vi "Drive Train Global.vi"() -> ()   [LabVIEW 2018]
panel:
  in  "Robot Slow Threshold":dbl=25.0
  in  "Robot Slow?":bool=TRUE
  in  "Robot Stopped?":bool=TRUE
  in  "Reset Field Position":bool
  in  "Wheel Angle Offsets Practice Bot":T1={"FrontLeft"=-114.2, "FrontRight"=-153.9, "BackLeft"=-23.0, "BackRight"=-19.1}
  in  "Angle Locking to":dbl=540.0
  in  "Angle to Lock To":dbl=180.0
  out "Lock to Angle":bool
  out "Robot Centric":bool
  in  "Don't Turn While Translate PID Gains":T2 {"derivative time (Td, min)" format="%.3f"; "integral time (Ti, min)" format="%.3f"; "proportional gain (Kc)" format="%.3f"}
  in  "Zero Yaw":bool
  in  "Wheel Angle Offsets":T1={"FrontLeft"=20.5, "FrontRight"=-178.8, "BackLeft"=-129.1, "BackRight"=-15.6}
  out "Wheel Angles":T1={"FrontLeft"=-0.09746133780628341, "FrontRight"=-0.37657886378471517, "BackLeft"=-0.0338013483928421, "BackRight"=0.42197930205392}
  in  "Rot. Point Y":dbl
  in  "Rot. Point X":dbl
  in  "Wheel Turn PID Values":T3={"Front Left"={"P Value"=0.014, "I Value"=0.0, "D Value"=0.0}, "Front Right"={"P Value"=0.014, "I Value"=0.0, "D Value"=0.0}, "Back Left"={"P Value"=0.014, "I Value"=0.0, "D Value"=0.0}, "Back Right"={"P Value"=0.014, "I Value"=0.0, "D Value"=0.0}}
  in  "Z Command":dbl=-0.02847923569553806
  in  "Y Command":dbl=-0.0
  out "Gyro Information":T4={"Rollover"=0.0, "Yaw"=-11.13, "Cont Yaw"=-11.13}
  in  "X Command":dbl
  in  "Current State":enum16{"Reached Position", "Going to Position"}(ring)
  in  "Current Mode":T5(ring)=enum."Field Oriented"
  out "Extra Info":bool
  out "Velocity":cluster{"X":dbl, "Y":dbl}
  out "Position":cluster{"X":dbl, "Y":dbl}={"X"=-0.530200643520846, "Y"=2.676204188026749}
  out "Wheel Drive Encoders":cluster{"Rates":dbl[], "Distances":dbl[]}={"Rates"=[0.0, 0.0, -0.0, -0.0], "Distances"=[-1.9909500000000002, 7.45781075, 7.561485, -2.9095839999999997]}
  # "X Command is spin"
  # "Z is X"
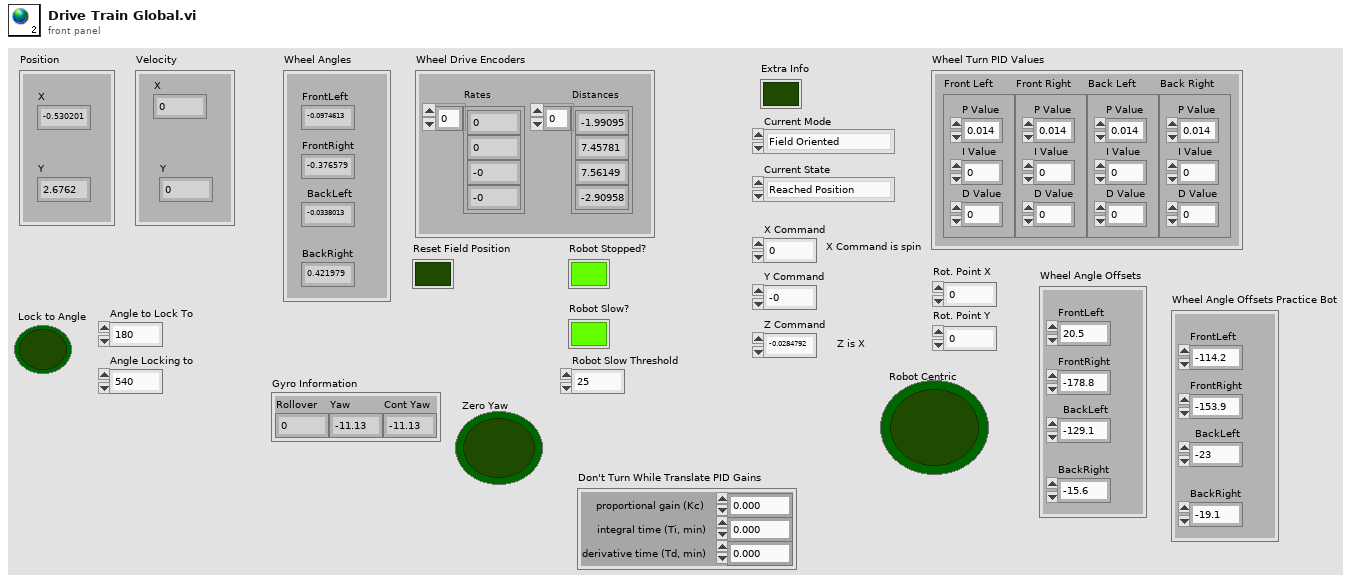
[diagram p1: front panel]
types:
  T1 = cluster{"FrontLeft":dbl, "FrontRight":dbl, "BackLeft":dbl, "BackRight":dbl}
  T2 = cluster{"proportional gain (Kc)":dbl, "integral time (Ti, min)":dbl, "derivative time (Td, min)":dbl}
  T3 = cluster{"Front Left":cluster{"P Value":dbl, "I Value":dbl, "D Value":dbl}, "Front Right":cluster{"P Value":dbl, "I Value":dbl, "D Value":dbl}, "Back Left":cluster{"P Value":dbl, "I Value":dbl, "D Value":dbl}, "Back Right":cluster{"P Value":dbl, "I Value":dbl, "D Value":dbl}}
  T4 = cluster{"Rollover":dbl, "Yaw":dbl, "Cont Yaw":dbl}
  T5 = enum16{"Autonomous Mode", "Field Oriented", "Robot Oriented", "Tank Mode"}
diagram:
